vi "ReadCalFile.vi"(0 "Wavelengths":dbl[](array[numeric])) -> (2 "file path out":path=path "Z:/Data/Old Data/Materials Testing/Calibration/2017-11-09/Multiplexter.tdms", 4 "Calibration Factor":dbl[](array[numeric]))   [LabVIEW 2018]
panel:
  in  "New Cal File?":bool
  out "Wavelengths":waveform(dbl)[](array[waveform])=[{"t0"=timestamp(0 s since 1904-01-01), "dt"=0.0, "Y"=array[2028 elements], "attributes"=variant("datatype"=variant(string "DT_DOUBLE"), "description"=variant(string ""), "displaytype"=variant(string "Numeric"), "monotony"=variant(string "not calculated"), "novaluekey"=variant(string "not calculated"))}, {"t0"=timestamp(0 s since 1904-01-01), "dt"=0.0, "Y"=array[512 elements], "attributes"=variant("datatype"=variant(string "DT_DOUBLE"), "description"=variant(string ""), "displaytype"=variant(string "Numeric"), "monotony"=variant(string "not calculated"), "novaluekey"=variant(string "not calculated"))}]
  out "Calibrations":waveform(dbl)[](array[waveform])=[{"t0"=timestamp(0 s since 1904-01-01), "dt"=0.0, "Y"=array[2028 elements], "attributes"=variant("datatype"=variant(string "DT_DOUBLE"), "description"=variant(string "Input: [7]/Radiance_Vis (514), [6]/Vis_Subtracted (511)"), "displaytype"=variant(string "Numeric"), "maximum"=variant(dbl 517.9862907743333), "minimum"=variant(dbl -541.6497859037797), "monotony"=variant(string "not monotone"), "novaluekey"=variant(string "Yes"))}, {"t0"=timestamp(0 s since 1904-01-01), "dt"=0.0, "Y"=array[512 elements], "attributes"=variant("datatype"=variant(string "DT_DOUBLE"), "description"=variant(string "Input: [7]/Radiance_NIR (515), [6]/NIR_Subtracted (512)"), "displaytype"=variant(string "Numeric"), "maximum"=variant(dbl 0.8399345575398146), "minimum"=variant(dbl 0.005655809178791624), "monotony"=variant(string "not monotone"), "novaluekey"=variant(string "Yes"))}]
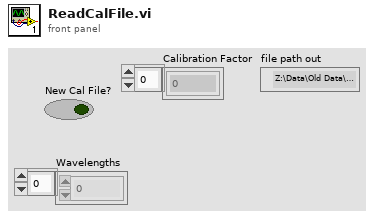
[diagram p1: front panel]
types:
  T1 = enum16{"open", "open or create", "create or replace", "create", "open (read-only)"}
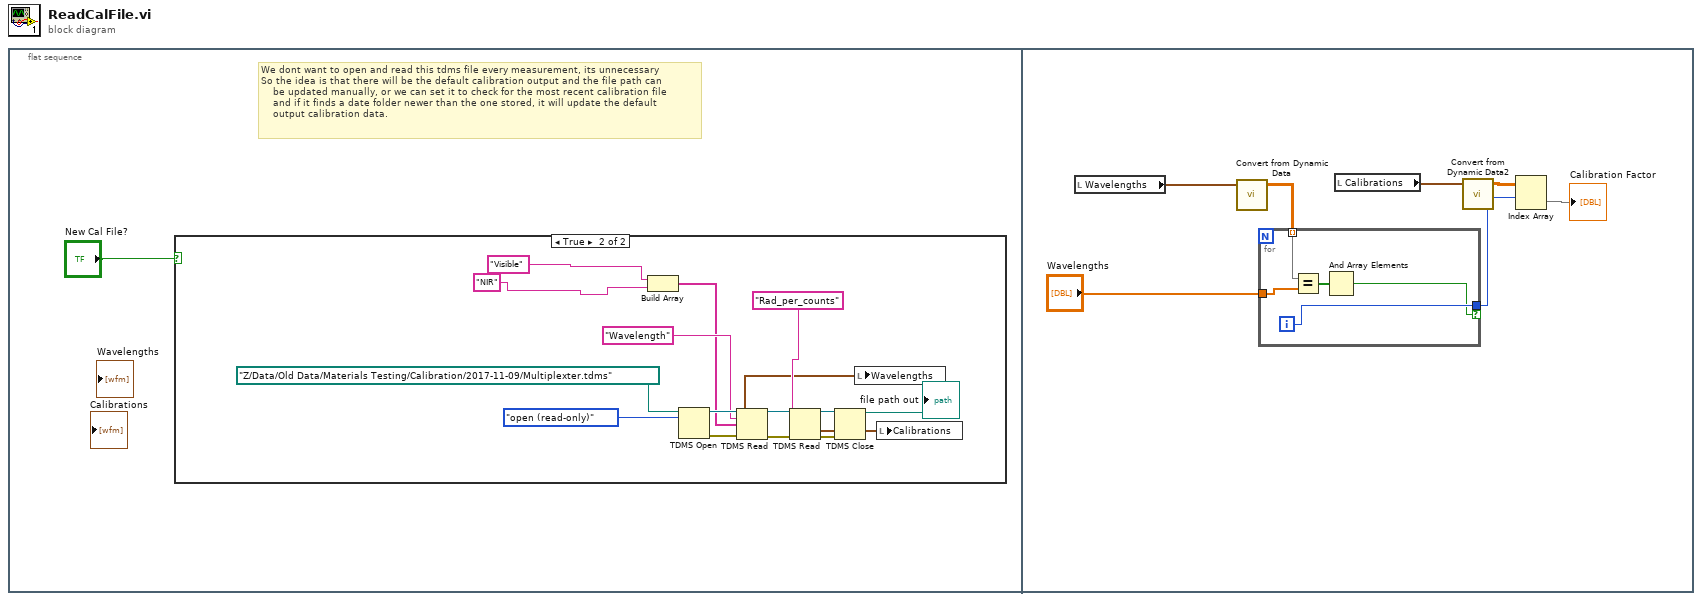
[diagram p0: block diagram]
diagram:
  n1 = flat-sequence {
    frame #0 {
      # "We dont want to open and read this tdms file every measurement, its unnecessary\nSo the idea is that there will be the default calibration output and the file path can \n    be updated manually, or we can set it to check for the most recent calibration file\n    and if it finds a date folder newer than the one stored, it will update the default \n    output calibration data."
      n2 = case shown="True" "New Cal File?" {
        frame False {
        }
        frame True {
          n3 = Build Array("Visible", "NIR") -> (w13:string[])
          n4 = TDMS Open(10:T1."open (read-only)" ("operation (0:open)"), 11:path "Z:/Data/Old Data/Materials Testing/Calibration/2017-11-09/Multiplexter.tdms" ("Normalization path")) -> (0:w15:errorcluster, 3:w16:refnum<k34>)  [unwired: 5 in]
          n5 = TDMS Read(0:w16, 5:"Wavelength" ("group name in"), 7:w13, 11:w15) -> (4:w12:refnum<k34>, 10:w5:waveform(dbl)[], 15:w11:errorcluster)  [unwired: 4 in, 3 out]
          n6 = TDMS Read(0:w12, 5:"Rad_per_counts", 11:w11) -> (4:w8:refnum<k34>, 10:w6:waveform(dbl)[], 15:w9:errorcluster)  [unwired: 5 in, 3 out]
          n7 = TDMS Close(8:w9, 11:w8) -> (3:→"file path out":path)  [unwired: 1 out]
          n8 = local write "Wavelengths"(w5) -> ()
          n9 = local write "Calibrations"(w6) -> ()
        }
      }
    }
    frame #1 {
      n10 = local read "Wavelengths"() -> (w19:waveform(dbl)[])
      n11 = call "Convert from Dynamic Data"("Dynamic Data Type"=w19) -> ("Array"=w20:dbl[][])  [unwired: 3 in]
      n12 = for {
        tunnel: "Wavelengths" -> [w29]
        tunnel: [w27] -> w21 if=w26
        tunnel: w20 -> [w25] mode=indexing
        i -> [w27]
        n13 = Equal?(x=w25, y=w29) -> (x = y?=w28:bool[])
        n14 = And Array Elements(Boolean array=w28) -> (logical AND=w26:bool)
      }
      n15 = local read "Calibrations"() -> (w24:waveform(dbl)[])
      n16 = call "Convert from Dynamic Data2"("Dynamic Data Type"=w24) -> ("Array"=w23:dbl[][])  [unwired: 3 in]
      n17 = Index Array(array=w23, index (row)=w21) -> (element=→"Calibration Factor":dbl[])  [unwired: 1 in]
    }
  }
